vi "LoadRegionbmp_171213.vi"(11 "SelectedPath":path) -> (3 "BackgroundSegmentforAnalysis":picture)   [LabVIEW 2016]
uses:
  Globaltracker.vi
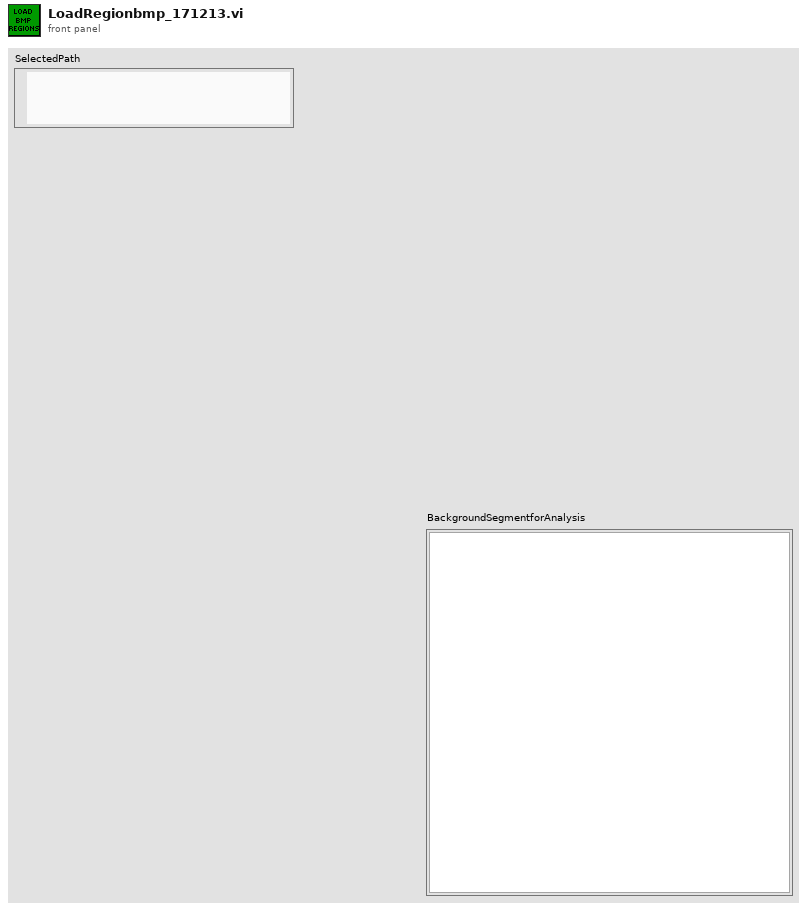
[diagram p1: front panel]
types:
  T1 = cluster{"left":i16, "top":i16, "right":i16, "bottom":i16}
  T2 = typedef "imagedata.ctl" = cluster{"image type":i32, "image depth":i32, "image":u8[], "mask":u8[], "colors":u32[], "Rectangle":cluster{"left":i16, "top":i16, "right":i16, "bottom":i16}}
  T3 = cluster{"image type":i32, "image depth":i32, "image":u8[], "mask":u8[], "colors":u32[], cluster{i32, i32, i32, i32}}
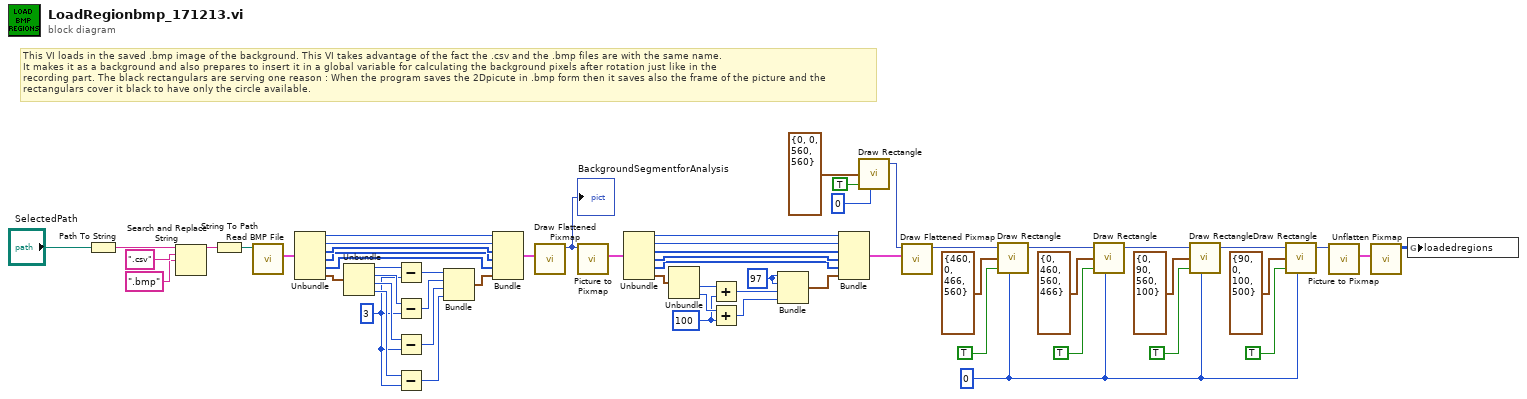
[diagram p0: block diagram]
diagram:
  w11 = 100
  w4 = 0
  w30 = 97
  w37 = 3
  # "This VI loads in the saved .bmp image of the background. This VI takes advantage of the fact the .csv and the .bmp files are with the same name.\nIt makes it as a background and also prepares to insert it in a global variable for calculating the background pixels after rotation just like in the\nrecording part. The black rectangulars are serving one reason : When the program saves the 2Dpicute in .bmp form then it saves also the frame of the picture and the \nrectangulars cover it black to have only the circle available."
  n1 = Path To String(path="SelectedPath") -> (string=w59:string)
  n2 = Search and Replace String(input string=w59, search string=".csv" ("substring (\"\")"), replace string=".bmp" ("replace string (\"\")")) -> (result string=w56:string)  [unwired: 5 in, 3 out]
  n3 = String To Path(string=w56) -> (path=w55:path)
  n4 = call <vilib>:"Read BMP File.vi"("path to BMP file"=w55) -> ("image data"=w54:T2)  [unwired: 8 in, 2 out]
  n5 = Unbundle(w54) -> ("image type"=w52:i32, "image depth"=w51:i32, "image"=w50:u8[], "mask"=w49:u8[], "colors"=w48:u32[], "Rectangle"=w53:T1)
  n6 = Unbundle(w53) -> ("left"=w45:i16, "top"=w40:i16, "right"=w39:i16, "bottom"=w38:i16)
  n7 = Subtract(x=w45, y=w37) -> (x-y=w44:i32)
  n8 = Subtract(x=w40, y=w37) -> (x-y=w43:i32)
  n9 = Subtract(x=w39, y=w37) -> (x-y=w42:i32)
  n10 = Subtract(x=w38, y=w37) -> (x-y=w41:i32)
  n11 = Bundle(w44, w43, w42, w41) -> (w47:cluster{i32, i32, i32, i32})  [unwired: 1 in]
  n12 = Bundle("image type"=w52, "image depth"=w51, "image"=w50, "mask"=w49, "colors"=w48, w47) -> (w46:T3)  [unwired: 1 in]
  n13 = call <vilib>:"Draw Flattened Pixmap.vi"("image data"=w46) -> ("new picture"=w12:picture)  [unwired: 8 in]
  "BackgroundSegmentforAnalysis" <- w12
  n14 = call <vilib>:"Picture to Pixmap.vi"("picture"=w12) -> ("image data"=w34:T2)  [unwired: 9 in, 1 out]
  n15 = Unbundle(w34) -> ("image type"=w27:i32, "image depth"=w26:i32, "image"=w25:u8[], "mask"=w24:u8[], "colors"=w23:u32[], "Rectangle"=w33:T1)
  n16 = Unbundle(w33) -> ("right"=w32:i16, "bottom"=w31:i16)  [unwired: 2 out]
  n17 = Add(x=w32, y=w11) -> (x+y=w29:i32)
  n18 = Add(x=w31, y=w11) -> (x+y=w28:i32)
  n19 = Bundle(w30, w30, w29, w28) -> (w22:cluster{i32, i32, i32, i32})  [unwired: 1 in]
  n20 = Bundle("image type"=w27, "image depth"=w26, "image"=w25, "mask"=w24, "colors"=w23, w22) -> (w21:T3)  [unwired: 1 in]
  n21 = call <vilib>:"Draw Rectangle.vi"("rect"=T1 {"left"=0, "top"=0, "right"=560, "bottom"=560}, "fill?(F)"=TRUE, "color(black)"=0) -> ("new picture"=w20:picture)  [unwired: 6 in]
  n22 = call <vilib>:"Draw Flattened Pixmap.vi"("image data"=w21, "picture"=w20) -> ("new picture"=w17:picture)  [unwired: 7 in]
  n23 = call <vilib>:"Draw Rectangle.vi"("picture"=w17, "rect"=T1 {"left"=460, "top"=0, "right"=466, "bottom"=560}, "fill?(F)"=TRUE, "color(black)"=w4) -> ("new picture"=w13:picture)  [unwired: 5 in]
  n24 = call <vilib>:"Draw Rectangle.vi"("picture"=w13, "rect"=T1 {"left"=0, "top"=460, "right"=560, "bottom"=466}, "fill?(F)"=TRUE, "color(black)"=w4) -> ("new picture"=w8:picture)  [unwired: 5 in]
  n25 = call <vilib>:"Draw Rectangle.vi"("picture"=w8, "rect"=T1 {"left"=0, "top"=90, "right"=560, "bottom"=100}, "fill?(F)"=TRUE, "color(black)"=w4) -> ("new picture"=w5:picture)  [unwired: 5 in]
  n26 = call <vilib>:"Draw Rectangle.vi"("picture"=w5, "rect"=T1 {"left"=90, "top"=0, "right"=100, "bottom"=500}, "fill?(F)"=TRUE, "color(black)"=w4) -> ("new picture"=w2:picture)  [unwired: 5 in]
  n27 = call <vilib>:"Picture to Pixmap.vi"("picture"=w2) -> ("image data"=w3:T2)  [unwired: 9 in, 1 out]
  n28 = call <vilib>:"Unflatten Pixmap.vi"("image data"=w3) -> ("24-bit pixmap"=w1:u32[][])  [unwired: 4 in, 6 out]
  n29 = global write "Globaltracker.vi" "loadedregions"(w1) -> ()
